vi "Set #Frames.vi"(8 "error in (no error)":errorcluster, 11 "CCDCamera in":refnum<class "CCDCamera.lvclass">) -> (0 "error out":errorcluster, 3 "CCDCamera out":refnum<class "CCDCamera.lvclass">)   [LabVIEW 2018, in "CCDCamera.lvclass"]
doc: "Set the number of frames in a kinetic series"
uses:
  CCDCamera.lvclass
  C:/Users/Denis/Desktop/S4ACS/SPARC4_ACS/Simulated_CCD_Camera/Simulated_CCD_Camera.lvclass
  Simulated_CCD_Camera/Simulated_CCD_Camera.lvclass
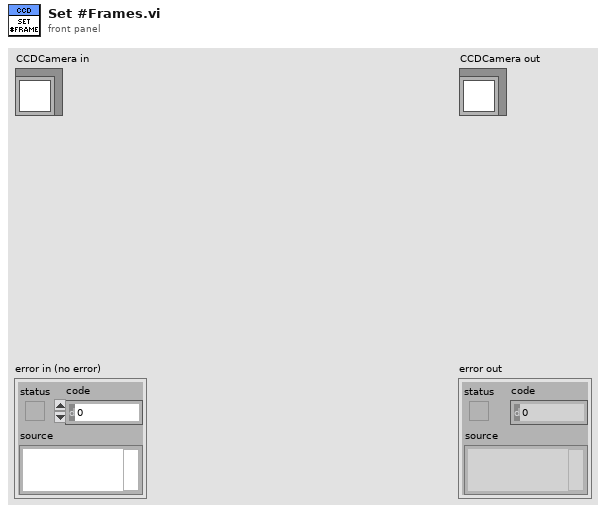
[diagram p1: front panel]
types:
  T1 = cluster{"COOLER_POWER_STATUS":u16, "TEMP":i32, "EXPTIME":dbl, "#FRAMES":u32, "#CYCLES":u32, "#SEQS":u32, "WAVEPLATE_POS":u16}
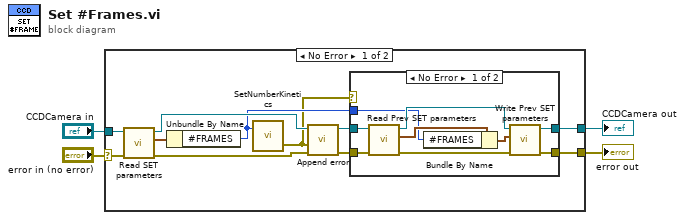
[diagram p0: block diagram]
diagram:
  n1 = case shown="No Error" "error in (no error)" {
    selector: "error in (no error)" -> [w15 w27]
    tunnel: "CCDCamera in" -> [w14 w28]
    tunnel: [w7 w27] -> w2
    tunnel: [w8 w28] -> w1
    frame No Error {
      n2 = call-dynamic "Read SET parameters.vi"("error in (no error)"=w15, "Simulated_CCD_Camera in"=w14) -> ("error out"=w13:errorcluster, "New SET parameters"=w12:T1, "Simulated_CCD_Camera out"=w11:refnum<class "CCDCamera.lvclass">)  [unwired: 7 in]
      n3 = Unbundle By Name(w12) -> ("#FRAMES"=w6:u32)
      n4 = call <userlib>:"SetNumberKinetics.vi"("number"=w6) -> ("error out"=w5:errorcluster)  [unwired: 1 in, 1 out]
      n5 = call "Append error.vi"("error in (no error)"=w13, "error"=w5, "Simulated_CCD_Camera in"=w11) -> ("error out"=w10:errorcluster, "Simulated_CCD_Camera out"=w9:refnum<class "CCDCamera.lvclass">)  [unwired: 7 in]
      n6 = case shown="No Error" w5 {
        tunnel: [w24 w26] -> w8
        tunnel: [w23 w25] -> w7
        tunnel: w9 -> [w19 w26]
        tunnel: w10 -> [w20 w25]
        tunnel: w6 -> [w16 _]
        frame No Error {
          n7 = call-dynamic "Read Prev SET parameters.vi"("error in (no error)"=w20, "Simulated_CCD_Camera in"=w19) -> ("error out"=w21:errorcluster, "Prev SET parameters"=w18:T1, "Simulated_CCD_Camera out"=w22:refnum<class "CCDCamera.lvclass">)  [unwired: 7 in]
          n8 = Bundle By Name(cluster=w18, "#FRAMES"=w16) -> (w17:T1)
          n9 = call-dynamic "Write Prev SET parameters.vi"("error in (no error)"=w21, "Prev SET parameters"=w17, "Simulated_CCD_Camera in"=w22) -> ("error out"=w23:errorcluster, "Simulated_CCD_Camera out"=w24:refnum<class "CCDCamera.lvclass">)  [unwired: 7 in]
        }
        frame Error {
        }
      }
    }
    frame Error {
    }
  }
  "error out" <- w2
  "CCDCamera out" <- w1
